vi "Edge Detection.vi"(8 "Error In":errorcluster, 10 "Blue Channel":T1(plugin-control), 11 "Red Channel":T1(plugin-control)) -> (0 "Error Out":errorcluster, 2 "Blue Edges":T1(plugin-control), 3 "Red Edges":T1(plugin-control))   [LabVIEW 2018]
uses:
  <vilib>/vision/NI_Vision_Development_Module.lvlib
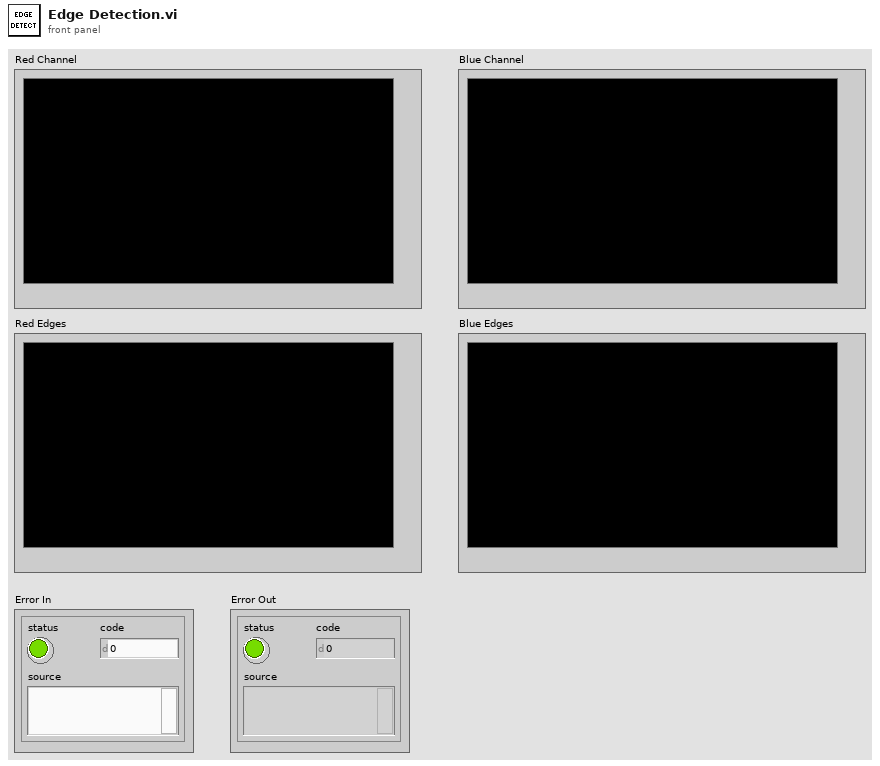
[diagram p1: front panel]
types:
  T1 = typedef "IMAQ Image.ctl" = refnum<image>
  T2 = cluster{"Sigma":sgl, "HThresh":sgl, "LThres":sgl, "WindowSize":i32}
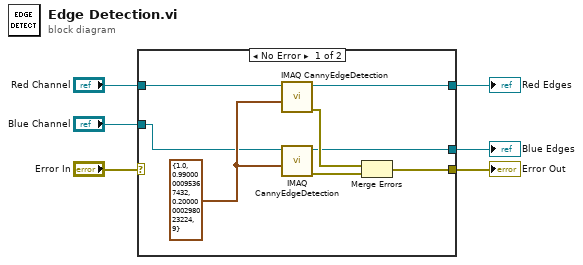
[diagram p0: block diagram]
diagram:
  n1 = case shown="No Error" "Error In" {
    selector: "Error In" -> [_ w17]
    tunnel: "Red Channel" -> [w12 w16]
    tunnel: "Blue Channel" -> [w13 w15]
    tunnel: [w9 w17] -> w2
    tunnel: [w8 w16] -> w3
    tunnel: [w7 w15] -> w1
    frame No Error {
      w14 = T2 {"Sigma"=1.0, "HThresh"=0.99, "LThres"=0.2, "WindowSize"=9} ("Filter Parameters")
      n2 = call "IMAQ CannyEdgeDetection"("Image Src"=w12, "Filter Parameters"=w14) -> ("Image Dst Out"=w8:T1, "error out"=w11:errorcluster)  [unwired: 6 in]
      n3 = call "IMAQ CannyEdgeDetection"("Image Src"=w13, "Filter Parameters"=w14) -> ("Image Dst Out"=w7:T1, "error out"=w10:errorcluster)  [unwired: 6 in]
      n4 = Merge Errors(w11, w10) -> (w9:errorcluster)
    }
    frame Error {
    }
  }
  "Error Out" <- w2
  "Red Edges" <- w3
  "Blue Edges" <- w1
